vi "Template.vi"() -> ()   [LabVIEW 2023]
panel:
  out "Vision Targets Found":bool
  out "Wrist On Target":bool
  out "Wrist Motor":dbl
  out "Wrist Position":dbl
  out "Wrist Setpoint":dbl
  out "Intake State":string
  out "Have Algae":bool
  out "Have Coral":bool
  out "Climb Position":dbl
  out "Climb Status":string
  out "Fully Pulled":bool
  out "Fully Reached":bool
  # "CLIMB"
  # "INTAKE"
  # "WRIST"
  # "VISION"
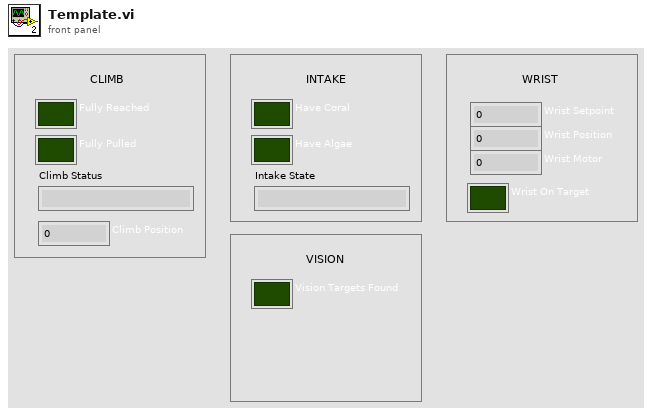
[diagram p1: front panel]
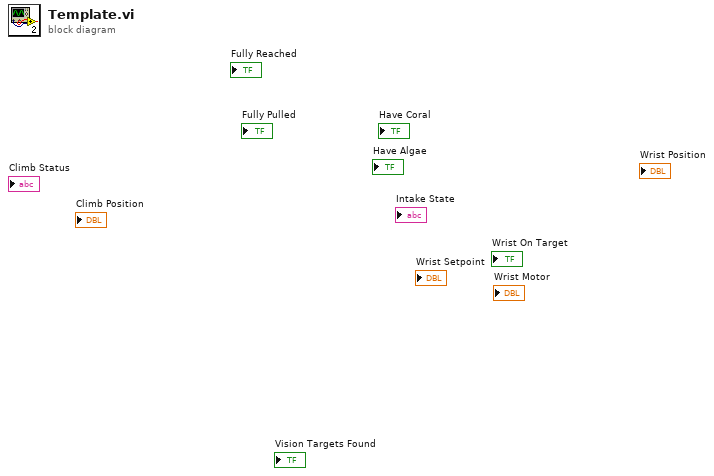
[diagram p0: block diagram]
diagram:
